vi "error.To JSON Tree.vi"(8 "error in (no error)":errorcluster, 11 "error in":refnum<class "error.lvclass">) -> (0 "error out":errorcluster, 2 "JSON Value out":variant, 3 "error out":refnum<class "error.lvclass">)   [LabVIEW 2017, in "error.lvclass"]
uses:
  error.lvclass
  error.lvclass/error.ctl
  <vilib>/National Instruments/Variant Data Manipulation/Insert Element at End.vi
  <vilib>/National Instruments/Variant Data Manipulation/Variant Data Manipulation.lvlib
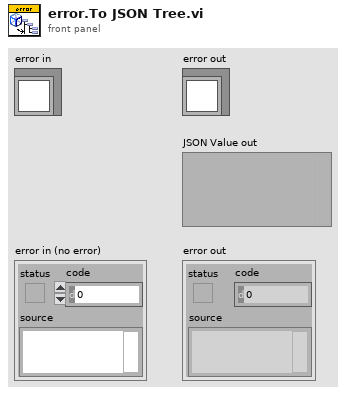
[diagram p1: front panel]
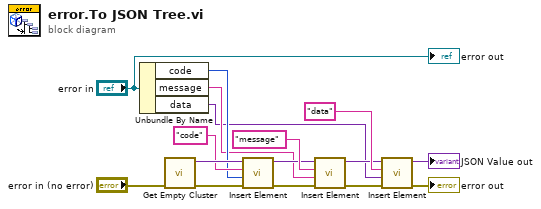
[diagram p0: block diagram]
diagram:
  n1 = Unbundle By Name("error in") -> ("code"=w13:i32, "message"=w10:string, "data"=w7:variant)
  n2 = call <vilib>:"Get Empty Cluster.vi"("error in (no error)"="error in (no error)") -> ("error out"=w6:errorcluster, "Variant (Cluster) out"=w15:variant)  [unwired: 9 in]
  n3 = call-poly <vilib>:"Insert Element.vi"("error in (no error)"=w6, "element"=w13, "Name"="code" ("Path in"), "Cluster in"=w15) -> ("error out"=w5:errorcluster, "Cluster out"=w11:variant)  [unwired: 6 in]
  n4 = call-poly <vilib>:"Insert Element.vi"("error in (no error)"=w5, "element"=w10, "Name"="message" ("Path in"), "Cluster in"=w11) -> ("error out"=w4:errorcluster, "Cluster out"=w8:variant)  [unwired: 6 in]
  n5 = call-poly <vilib>:"Insert Element.vi"("error in (no error)"=w4, "element"=w7, "Name"="data" ("Path in"), "Cluster in"=w8) -> ("error out"=→"error out":errorcluster, "Cluster out"=→"JSON Value out":variant)  [unwired: 6 in]
  "error out" <- "error in"
